vi "SigmaDeltaModulator.vi"(6 "Coef.c":dbl[](array[numeric]), 8 "Coef.b":dbl[](array[numeric]), 9 "FeedbackVal":dbl, 10 "Coef.a":dbl[](array[numeric]), 11 "InputData":dbl[](array[numeric])) -> (3 "OutputData":dbl[][](array[numeric]))   [LabVIEW 2016]
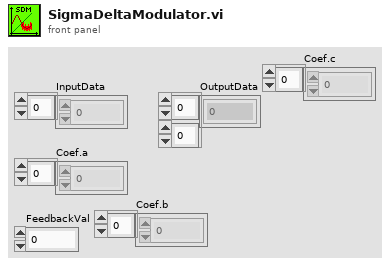
[diagram p1: front panel]
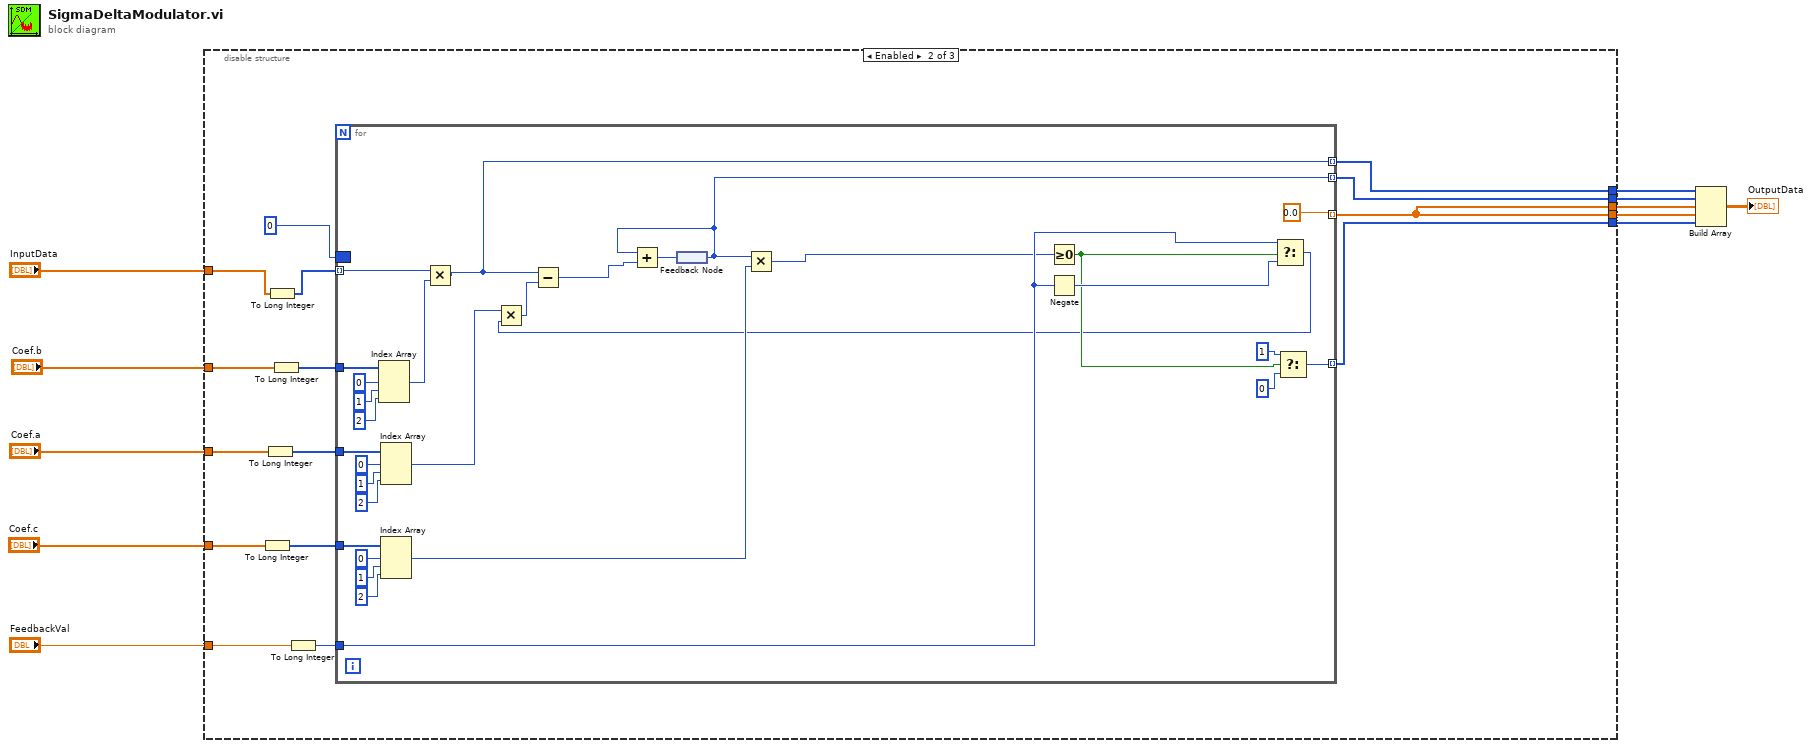
[diagram p0: block diagram]
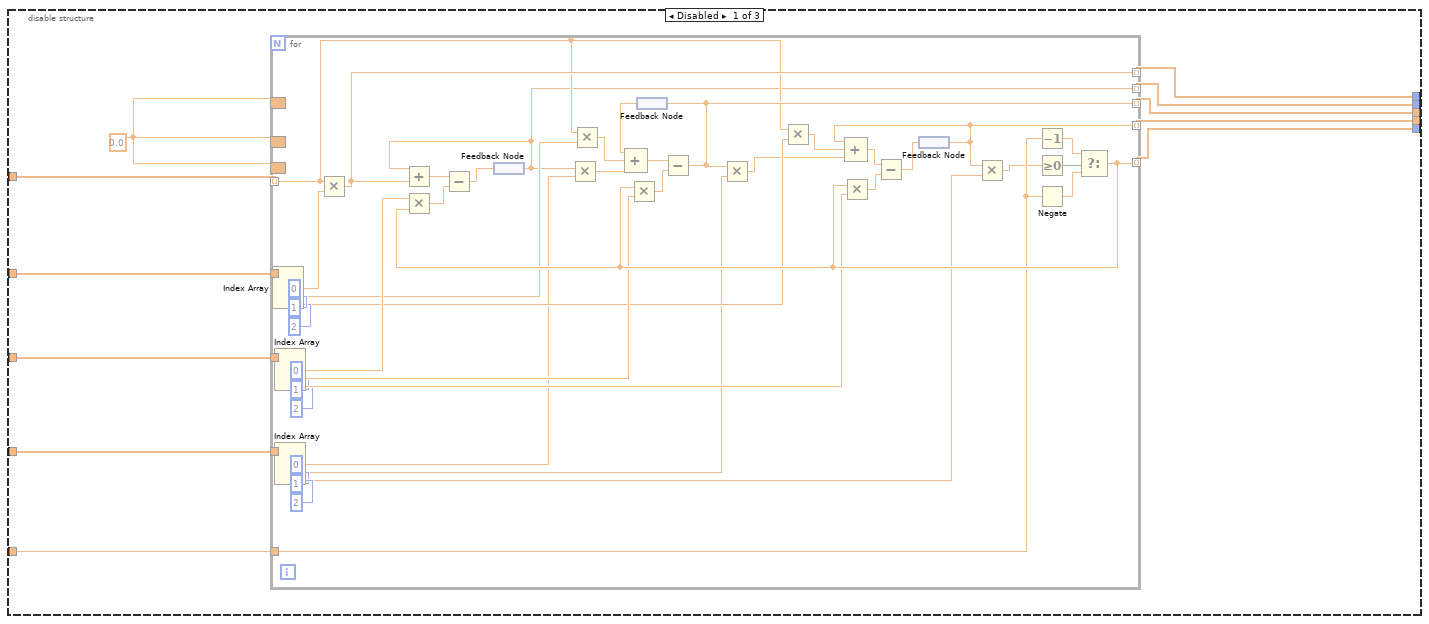
[diagram p2: hidden frame]
diagram:
  n1 = disable-structure shown="Enabled" {
    disable-tunnel: "FeedbackVal" -> [w22 w77 _]
    disable-tunnel: "Coef.a" -> [w21 w82 _]
    disable-tunnel: "InputData" -> [w19 w75 _]
    disable-tunnel: [w18 w69 _] -> w8
    disable-tunnel: [w17 w78 _] -> w7
    disable-tunnel: [w16 w78 _] -> w6
    disable-tunnel: [w15 w76 _] -> w5
    disable-tunnel: [w14 w81 _] -> w4
    disable-tunnel: "Coef.b" -> [w13 w80 _]
    disable-tunnel: "Coef.c" -> [w12 w79 _]
    frame Disabled {
      w20 = 0.0
      n2 = for {
        tunnel: w19 -> [w35] mode=indexing
        tunnel: [w36] -> w17 mode=indexing
        tunnel: [w58] -> w18 mode=indexing
        tunnel: [w49] -> w14 mode=indexing
        tunnel: [w29] -> w15 mode=indexing
        tunnel: [w38] -> w16 mode=indexing
        border: w20 -> [_]
        border: w20 -> [_]
        border: w20 -> [_]
        tunnel: w21 -> [w57]
        tunnel: w22 -> [w50]
        tunnel: w13 -> [w45]
        tunnel: w12 -> [w30]
        n3 = Index Array(array=w45, index #1=0 ("index"), index #2=1 ("index"), index #3=2 ("index")) -> (element #1=w44:dbl, element #2=w40:dbl, element #3=w34:dbl)
        n4 = Index Array(array=w57, index #1=0 ("index"), index #2=1 ("index"), index #3=2 ("index")) -> (element #1=w56:dbl, element #2=w54:dbl, element #3=w53:dbl)
        n5 = Index Array(array=w30, index #1=0 ("index"), index #2=1 ("index"), index #3=2 ("index")) -> (element #1=w27:dbl, element #2=w25:dbl, element #3=w23:dbl)
        n6 = Multiply(x=w35, y=w44) -> (x*y=w49:dbl)
        n7 = feedback #1() -> (w29:dbl)
        n8 = Add(x=w29, y=w49) -> (x+y=w67:dbl)
        n9 = Multiply(x=w29, y=w27) -> (x*y=w28:dbl)
        n10 = Multiply(x=w35, y=w40) -> (x*y=w41:dbl)
        n11 = feedback #2() -> (w43:dbl)
        n12 = Compound Arithmetic op=ADD(w43, w41, w28) -> (w42:dbl)
        n13 = Multiply(x=w35, y=w34) -> (x*y=w39:dbl)
        n14 = feedback #3() -> (w36:dbl)
        n15 = Multiply(x=w36, y=w23) -> (x*y=w24:dbl)
        n16 = Decrement(x=w50) -> (x-1=w62:dbl)
        n17 = Greater Or Equal To 0?(x=w24) -> (x >= 0?=w63:bool)
        n18 = Negate(x=w50) -> (-x=w61:dbl)
        n19 = Select(t=w62, s=w63, f=w61) -> (s? t:f=w58:dbl)
        n20 = Multiply(x=w56, y=w58) -> (x*y=w64:dbl)
        n21 = Subtract(x=w67, y=w64) -> (x-y=w66:dbl)
        n22 = feedback-in #1(w66) -> ()
        n23 = Multiply(x=w58, y=w54) -> (x*y=w65:dbl)
        n24 = Subtract(x=w42, y=w65) -> (x-y=w38:dbl)
        n25 = feedback-in #2(w38) -> ()
        n26 = Multiply(x=w38, y=w25) -> (x*y=w26:dbl)
        n27 = Multiply(x=w58, y=w53) -> (x*y=w60:dbl)
        n28 = Compound Arithmetic op=ADD(w36, w39, w26) -> (w37:dbl)
        n29 = Subtract(x=w37, y=w60) -> (x-y=w59:dbl)
        n30 = feedback-in #3(w59) -> ()
      }
    }
    frame Enabled {
      n31 = To Long Integer(number=w79) -> (32bit integer=w71:i32[])
      n32 = To Long Integer(number=w82) -> (32bit integer=w72:i32[])
      n33 = To Long Integer(number=w75) -> (32bit integer=w74:i32[])
      n34 = To Long Integer(number=w80) -> (32bit integer=w73:i32[])
      n35 = To Long Integer(number=w77) -> (32bit integer=w70:i32)
      n36 = for {
        tunnel: w74 -> [w100] mode=indexing
        tunnel: [w85] -> w81 mode=indexing
        tunnel: [w88] -> w76 mode=indexing
        border: 0 -> [_]
        tunnel: w72 -> [w111]
        tunnel: w70 -> [w106]
        tunnel: w73 -> [w102]
        tunnel: w71 -> [w96]
        tunnel: [0.0] -> w78 mode=indexing
        tunnel: [w90] -> w69 mode=indexing
        n37 = Index Array(array=w102, index #1=0 ("index"), index #2=1 ("index"), index #3=2 ("index")) -> (element #1=w101:i32)  [unwired: 2 out]
        n38 = Index Array(array=w111, index #1=0 ("index"), index #2=1 ("index"), index #3=2 ("index")) -> (element #1=w110:i32)  [unwired: 2 out]
        n39 = Index Array(array=w96, index #1=0 ("index"), index #2=1 ("index"), index #3=2 ("index")) -> (element #1=w95:i32)  [unwired: 2 out]
        n40 = Multiply(x=w100, y=w101) -> (x*y=w85:i32)
        n41 = feedback #4() -> (w88:i32)
        n42 = Multiply(x=w88, y=w95) -> (x*y=w86:i32)
        n43 = Greater Or Equal To 0?(x=w86) -> (x >= 0?=w93:bool)
        n44 = Negate(x=w106) -> (-x=w112:i32)
        n45 = Select(t=w106, s=w93, f=w112) -> (s? t:f=w83:i32)
        n46 = Multiply(x=w110, y=w83) -> (x*y=w87:i32)
        n47 = Subtract(x=w85, y=w87) -> (x-y=w84:i32)
        n48 = Add(x=w88, y=w84) -> (x+y=w89:i32)
        n49 = feedback-in #4(w89) -> ()
        n50 = Select(t=1 ("s? t:f"), s=w93, f=0 ("s? t:f")) -> (s? t:f=w90:i32)
      }
    }
    frame Disabled {
    }
  }
  n51 = Build Array(w4, w5, w6, w7, w8) -> (→"OutputData":dbl[][])
